vi "Lightning Drive Train.vi"(8 "error in (no error)":errorcluster, 10 "Enum":T1, 11 "Refnum in":refnum<k33>) -> ()   [LabVIEW 2013]
uses:
  Drive Train States.ctl
  dashboard/TeleopCmd.ctl
  CmdFlag.ctl
  <vilib>/Rock Robotics/WPI/Solenoid/WPI_SolenoidValue.ctl
  <vilib>/Rock Robotics/WPI/Solenoid/WPI_SolenoidGetEnum.vi
  <vilib>/Rock Robotics/WPI/Solenoid/WPI_SolenoidSetEnum.vi
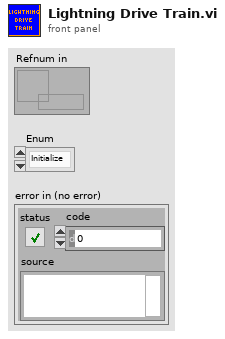
[diagram p1: front panel]
types:
  T1 = typedef "Drive Train States.ctl" = enum16{"Initialize", "Low_gear", "Upshift", "Wait For Upshift", "Upshift Complete", "High_gear", "Downshift", "Wait For Downshift", "Downshift Complete", "Suspend", "Resume"}
  T2 = typedef "WPI_SolenoidValue.ctl" = enum16{"Off", "On", "Forward", "Reverse"}
  T3 = typedef "WPI_SolenoidDevRef.ctl" = cluster{"DevStatus":errorcluster, "Solenoid Module":T4, "Forward Solenoid Channel":T5, "Reverse Solenoid Channel":T5}
  T4 = typedef "FPGA_TypedefSolenoidModule.ctl" = enum16{"Solenoid Module 1", "Solenoid Module 2"}
  T5 = typedef "WPI_SolenoidChannel.ctl" = enum8{"Solenoid 1", "Solenoid 2", "Solenoid 3", "Solenoid 4", "Solenoid 5", "Solenoid 6", "Solenoid 7", "Solenoid 8", "Invalid"}
  T6 = typedef "TeleopCmd.ctl" = cluster{"Left Joystick":dbl, "Right Joystick":dbl, "Shift":bool, "CmdFlag":T7}
  T7 = typedef "CmdFlag.ctl" = enum16{"noop", "suspend", "resume"}
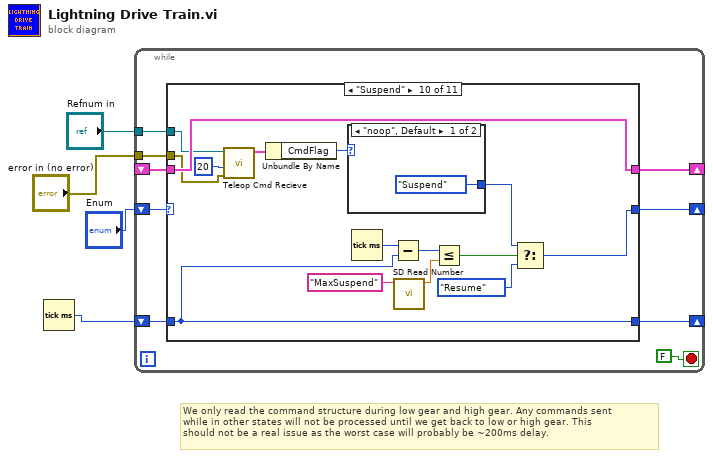
[diagram p0: block diagram]
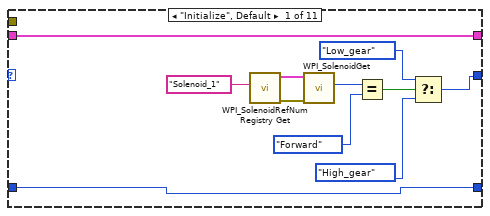
[diagram p2: hidden frame]
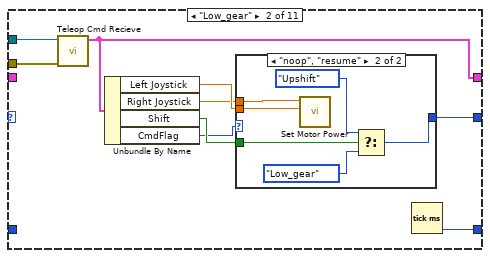
[diagram p3: hidden frame]
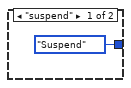
[diagram p4: hidden frame]
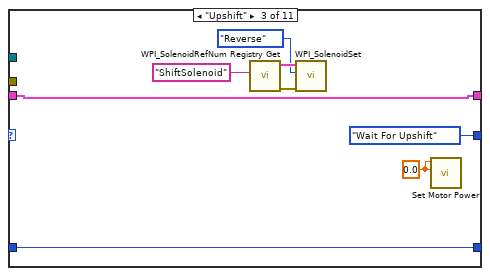
[diagram p5: hidden frame]
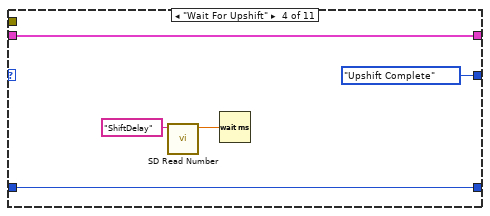
[diagram p6: hidden frame]
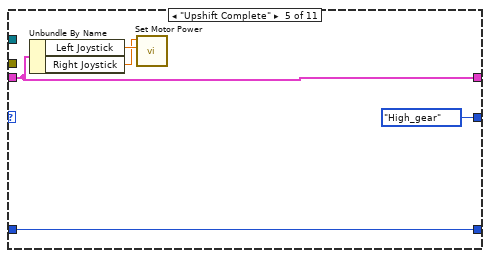
[diagram p7: hidden frame]
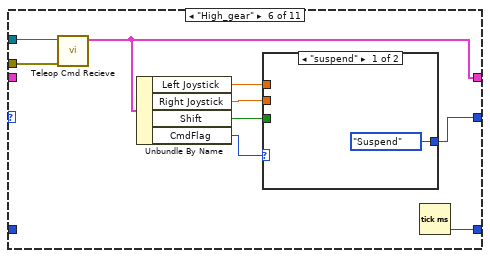
[diagram p8: hidden frame]
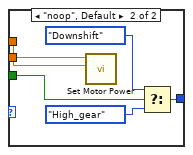
[diagram p9: hidden frame]
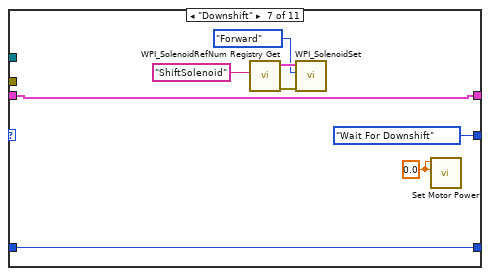
[diagram p10: hidden frame]
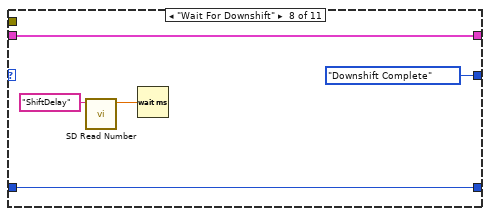
[diagram p11: hidden frame]
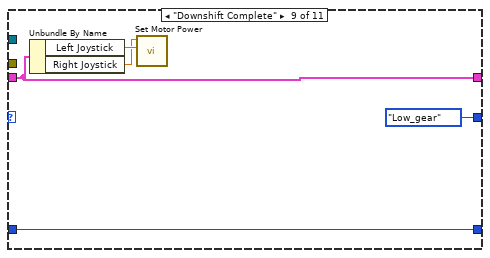
[diagram p12: hidden frame]
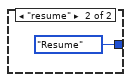
[diagram p13: hidden frame]
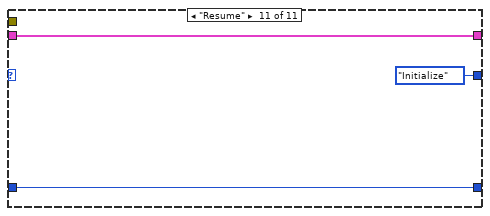
[diagram p14: hidden frame]
diagram:
  # "We only read the command structure during low gear and high gear. Any commands sent\nwhile in other states will not be processed until we get back to low or high gear. This \nshould not be a real issue as the worst case will probably be ~200ms delay."
  n1 = Tick Count (ms)() -> (millisecond timer value=w1:u32)
  n2 = while {
    tunnel: "Refnum in" -> [w12]
    tunnel: "error in (no error)" -> [w11]
    shift-right: [w7] -> _
    shift-left: "Enum" -> [w10]
    shift-right: [w9] -> _
    shift-left: _ -> [w8]
    shift-right: [w6] -> _
    shift-left: w1 -> [w5]
    stop <- FALSE stop-if-true
    n3 = case shown="\"Suspend\"" w10 {
      tunnel: w12 -> [_ w33 _ _ _ w67 _ _ _ w104 _]
      tunnel: w11 -> [_ w32 _ _ _ w66 _ _ _ w105 _]
      tunnel: [w16 w30 Drive_Train_States."Wait For Upshift" Drive_Train_States."Upshift Complete" Drive_Train_States."High_gear" w63 Drive_Train_States."Wait For Downshift" Drive_Train_States."Downshift Complete" Drive_Train_States."Low_gear" w93 Drive_Train_States."Initialize"] -> w7
      tunnel: [w15 w29 w43 w52 w57 w65 w78 w86 w91 w107 w112] -> w9
      tunnel: w8 -> [w15 _ w43 w52 w57 _ w78 w86 w91 w107 w112]
      tunnel: w5 -> [w14 _ w41 w49 w54 _ w75 w83 w88 w99 w110]
      tunnel: [w14 w25 w41 w49 w54 w60 w75 w83 w88 w99 w110] -> w6
      frame "Initialize", Default {
        n4 = call <vilib>:"WPI_SolenoidRefNum Registry Get.vi"("refnum name"="Solenoid_1") -> ("error out"=w24:errorcluster, "SolenoidDevRef"=w23:T3)  [unwired: 9 in]
        n5 = call-poly <vilib>:"WPI_SolenoidGet.vi"("error in (no error)"=w24, "SolenoidDevRef"=w23) -> ("Value"=w21:T2)  [unwired: 7 in, 2 out]
        n6 = Equal?(x=w21, y=WPI_SolenoidValue."Forward") -> (x = y?=w19:bool)
        n7 = Select(t=Drive_Train_States."Low_gear", s=w19, f=Drive_Train_States."High_gear") -> (s? t:f=w16:T1)
      }
      frame "Low_gear" {
        n8 = call "Teleop Cmd Recieve.vi"("error in (no error)"=w32, "rt fifo"=w33) -> ("element out"=w29:T6)  [unwired: 8 in, 1 out]
        n9 = Unbundle By Name(w29) -> ("Left Joystick"=w28:dbl, "Right Joystick"=w27:dbl, "Shift"=w31:bool, "CmdFlag"=w26:T7)
        n10 = case shown="\"noop\", \"resume\"" w26 {
          tunnel: w31 -> [_ w40]
          tunnel: [Drive_Train_States."Suspend" w37] -> w30
          tunnel: w28 -> [_ w36]
          tunnel: w27 -> [_ w35]
          frame "suspend" {
          }
          frame "noop", "resume" {
            n11 = call "Set Motor Power.vi"("Left Motor Power"=w36, "Right Motor Power"=w35) -> ()  [unwired: 10 in]
            n12 = Select(t=Drive_Train_States."Upshift", s=w40, f=Drive_Train_States."Low_gear") -> (s? t:f=w37:T1)
          }
        }
        n13 = Tick Count (ms)() -> (millisecond timer value=w25:u32)
      }
      frame "Upshift" {
        w42 = 0.0 ("Output")
        n14 = call <vilib>:"WPI_SolenoidRefNum Registry Get.vi"("refnum name"="ShiftSolenoid") -> ("error out"=w48:errorcluster, "SolenoidDevRef"=w47:T3)  [unwired: 9 in]
        n15 = call-poly <vilib>:"WPI_SolenoidSet.vi"("error in (no error)"=w48, "Value"=WPI_SolenoidValue."Reverse", "SolenoidDevRef"=w47) -> ()  [unwired: 7 in, 2 out]
        n16 = call "Set Motor Power.vi"("Left Motor Power"=w42, "Right Motor Power"=w42) -> ()  [unwired: 10 in]
      }
      frame "Wait For Upshift" {
        n17 = call <vilib>:"SD Read Number.vi"("Name"="ShiftDelay") -> ("Numeric"=w50:dbl)  [unwired: 8 in, 2 out]
        n18 = Wait (ms)(milliseconds to wait=w50) -> ()  [unwired: 1 out]
      }
      frame "Upshift Complete" {
        n19 = Unbundle By Name(w57) -> ("Left Joystick"=w56:dbl, "Right Joystick"=w55:dbl)
        n20 = call "Set Motor Power.vi"("Left Motor Power"=w56, "Right Motor Power"=w55) -> ()  [unwired: 10 in]
      }
      frame "High_gear" {
        n21 = call "Teleop Cmd Recieve.vi"("error in (no error)"=w66, "rt fifo"=w67) -> ("element out"=w65:T6)  [unwired: 8 in, 1 out]
        n22 = Unbundle By Name(w65) -> ("Left Joystick"=w62:dbl, "Right Joystick"=w61:dbl, "Shift"=w64:bool, "CmdFlag"=w59:T7)
        n23 = case shown="\"suspend\"" w59 {
          tunnel: w64 -> [_ w72]
          tunnel: [Drive_Train_States."Suspend" w71] -> w63
          tunnel: w62 -> [_ w70]
          tunnel: w61 -> [_ w69]
          frame "suspend" {
          }
          frame "noop", Default {
            n24 = call "Set Motor Power.vi"("Left Motor Power"=w70, "Right Motor Power"=w69) -> ()  [unwired: 10 in]
            n25 = Select(t=Drive_Train_States."Downshift", s=w72, f=Drive_Train_States."High_gear") -> (s? t:f=w71:T1)
          }
        }
        n26 = Tick Count (ms)() -> (millisecond timer value=w60:u32)
      }
      frame "Downshift" {
        w76 = 0.0 ("Output")
        n27 = call <vilib>:"WPI_SolenoidRefNum Registry Get.vi"("refnum name"="ShiftSolenoid") -> ("error out"=w82:errorcluster, "SolenoidDevRef"=w81:T3)  [unwired: 9 in]
        n28 = call-poly <vilib>:"WPI_SolenoidSet.vi"("error in (no error)"=w82, "Value"=WPI_SolenoidValue."Forward", "SolenoidDevRef"=w81) -> ()  [unwired: 7 in, 2 out]
        n29 = call "Set Motor Power.vi"("Left Motor Power"=w76, "Right Motor Power"=w76) -> ()  [unwired: 10 in]
      }
      frame "Wait For Downshift" {
        n30 = call <vilib>:"SD Read Number.vi"("Name"="ShiftDelay") -> ("Numeric"=w84:dbl)  [unwired: 8 in, 2 out]
        n31 = Wait (ms)(milliseconds to wait=w84) -> ()  [unwired: 1 out]
      }
      frame "Downshift Complete" {
        n32 = Unbundle By Name(w91) -> ("Left Joystick"=w90:dbl, "Right Joystick"=w89:dbl)
        n33 = call "Set Motor Power.vi"("Left Motor Power"=w90, "Right Motor Power"=w89) -> ()  [unwired: 10 in]
      }
      frame "Suspend" {
        n34 = call "Teleop Cmd Recieve.vi"("error in (no error)"=w105, "timeout in ms (0)"=20, "rt fifo"=w104) -> ("element out"=w106:T6)  [unwired: 7 in, 1 out]
        n35 = Unbundle By Name(w106) -> ("CmdFlag"=w103:T7)
        n36 = case shown="\"noop\", Default" w103 {
          tunnel: [Drive_Train_States."Suspend" Drive_Train_States."Resume"] -> w94
          frame "noop", Default {
          }
          frame "resume" {
          }
        }
        n37 = Tick Count (ms)() -> (millisecond timer value=w100:u32)
        n38 = Subtract(x=w100, y=w99) -> (x-y=w98:u32)
        n39 = call <vilib>:"SD Read Number.vi"("Name"="MaxSuspend") -> ("Numeric"=w97:dbl)  [unwired: 8 in, 2 out]
        n40 = Less Or Equal?(x=w98, y=w97) -> (x <= y?=w96:bool)
        n41 = Select(t=w94, s=w96, f=Drive_Train_States."Resume") -> (s? t:f=w93:T1)
      }
      frame "Resume" {
      }
    }
  }
